vi "ROI group-Event handler-Shortcut menu activ.vi"(9 "Coords":T1, 11 "[Groups] menu ref":refnum<k9>) -> (0 "error out":errorcluster)   [LabVIEW 2020]
uses:
  <vilib>/Utility/miscctls.llb/LVPoint32TypeDef.ctl
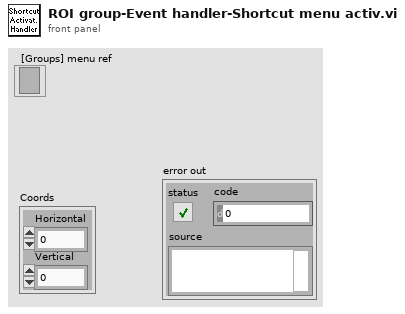
[diagram p1: front panel]
types:
  T1 = typedef "LVPoint32TypeDef.ctl" = cluster{"Horizontal":i32, "Vertical":i32}
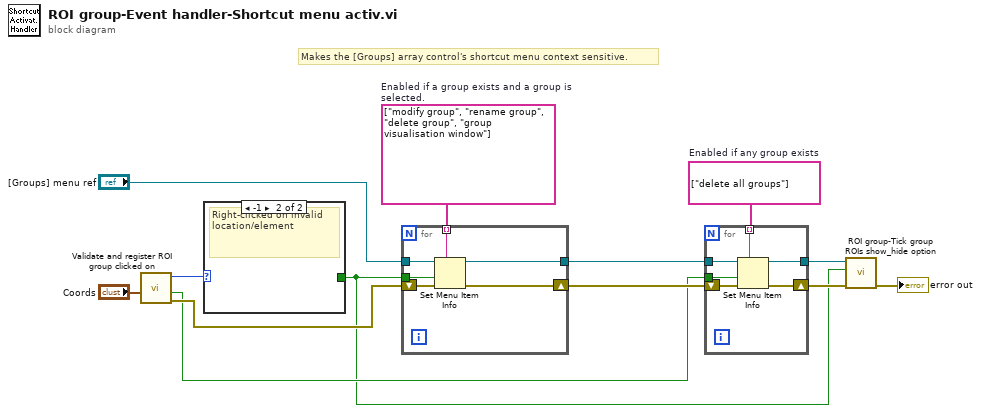
[diagram p0: block diagram]
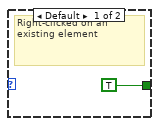
[diagram p2: hidden frame]
diagram:
  w10 = string[] ["delete all groups"]  # Enabled if any group exists
  w11 = string[] ["modify group", "rename group", "delete group", "group visualisation window"]  # Enabled if a group exists and a group is selected.
  # "Makes the [Groups] array control's shortcut menu context sensitive."
  n1 = call "Validate and register ROI group clicked on.vi"("Coords"="Coords") -> ("error out"=w6:errorcluster, "Array is not empty"=w2:bool, "Index of group clicked on"=w12:i16)  [unwired: 8 in]
  n2 = case shown="-1" w12 {
    tunnel: [TRUE _] -> w1
    frame Default {
      # "Right-clicked on an existing element"
    }
    frame -1 {
      # "Right-clicked on invalid location/element"
    }
  }
  n3 = for {
    tunnel: "[Groups] menu ref" -> [w20]
    tunnel: w11 -> [w19] mode=indexing
    tunnel: w1 -> [w18]
    tunnel: [w17] -> w9
    shift-right: [w15] -> w8
    shift-left: w6 -> [w16]
    n4 = Set Menu Item Info(7:w19, 8:w16, 9:w18, 11:w20) -> (0:w15:errorcluster, 3:w17:refnum<k9>)  [unwired: 3 in]
  }
  n5 = for {
    tunnel: w9 -> [w26]
    tunnel: w10 -> [w25] mode=indexing
    tunnel: w2 -> [w24]
    shift-right: [w22] -> w5
    shift-left: w8 -> [w23]
    tunnel: [w21] -> w3
    n6 = Set Menu Item Info(7:w25, 8:w23, 9:w24, 11:w26) -> (0:w22:errorcluster, 3:w21:refnum<k9>)  [unwired: 3 in]
  }
  n7 = call "ROI group-Tick group ROIs show_hide option.vi"("error in (no error)"=w5, "Valid?"=w1, "Menu in"=w3) -> ("error out"=→"error out":errorcluster)  [unwired: 7 in, 1 out]
